vi "Write Start Command notifier.vi"(8 "error in (no error)":errorcluster, 10 "Start Command notifier":refnum<notifier>, 11 "Command Actor in":refnum<class "Command Actor.lvclass">) -> (0 "error out":errorcluster, 3 "Command Actor out":refnum<class "Command Actor.lvclass">)   [LabVIEW 2014, in "Robot Actor Framework.lvlib" / "Command Actor.lvlib" / "Command Actor.lvclass"]
uses:
  Command Actor.lvclass
  Command Actor.lvclass/Command Actor.ctl
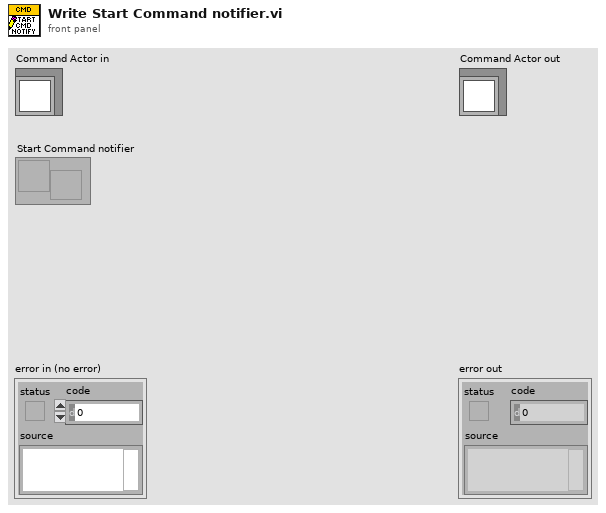
[diagram p1: front panel]
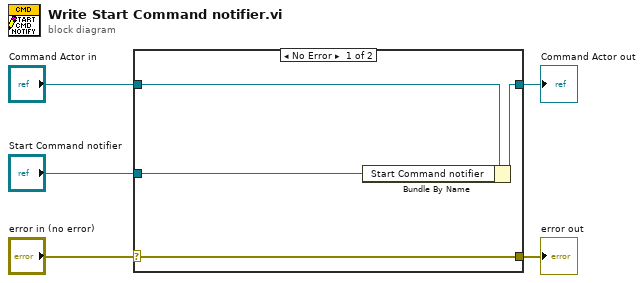
[diagram p0: block diagram]
diagram:
  n1 = case shown="No Error" "error in (no error)" {
    selector: "error in (no error)" -> [w9 w10]
    tunnel: [w9 w10] -> w4
    tunnel: [w7 w11] -> w2
    tunnel: "Command Actor in" -> [w8 w11]
    tunnel: "Start Command notifier" -> [w6 _]
    frame No Error {
      n2 = Bundle By Name(cluster=w8, "Start Command notifier"=w6) -> (w7:refnum<class "Command Actor.lvclass">)
    }
    frame Error {
    }
  }
  "error out" <- w4
  "Command Actor out" <- w2
